vi "Add Channel.vi"(7 "Display State In":T1={"Current Channels Info"=[], "Help Prefix"="", "Max Display Size"=8, "Max Size"=0, "Show Buttons"=TRUE, "Data Valid"=refnum, "Show Range"=FALSE, "Range Items"=[], "Range Index"=[]}, 11 "Channels In":T4) -> (3 "Channels Out":T4, 5 "Display State Out":T1={"Current Channels Info"=[], "Help Prefix"="", "Max Display Size"=8, "Max Size"=0, "Show Buttons"=TRUE, "Data Valid"=refnum, "Show Range"=FALSE, "Range Items"=[], "Range Index"=[]})   [LabVIEW 2021, in "myRIO Channel List.xctl"]
uses:
  <vilib>/myRIO/Common/Express VI Framework/xctls/myRIO Channel List/myRIO Channel List.xctl
  <vilib>/myRIO/Common/Express VI Framework/xctls/myRIO Channel List/Data.ctl
  <vilib>/myRIO/Common/Express VI Framework/xctls/myRIO Channel List/typedefs/Channel Data.ctl
  <vilib>/myRIO/Common/Express VI Framework/xctls/myRIO Channel List/typedefs/Remove Channel.ctl
  <vilib>/myRIO/Common/Express VI Framework/xctls/myRIO Channel List/State.ctl
  <vilib>/myRIO/Common/Profile Manager Framework/typedefs/Channel Info.ctl
  <vilib>/myRIO/Common/Express VI Framework/typedefs/Data Validate Ref.ctl
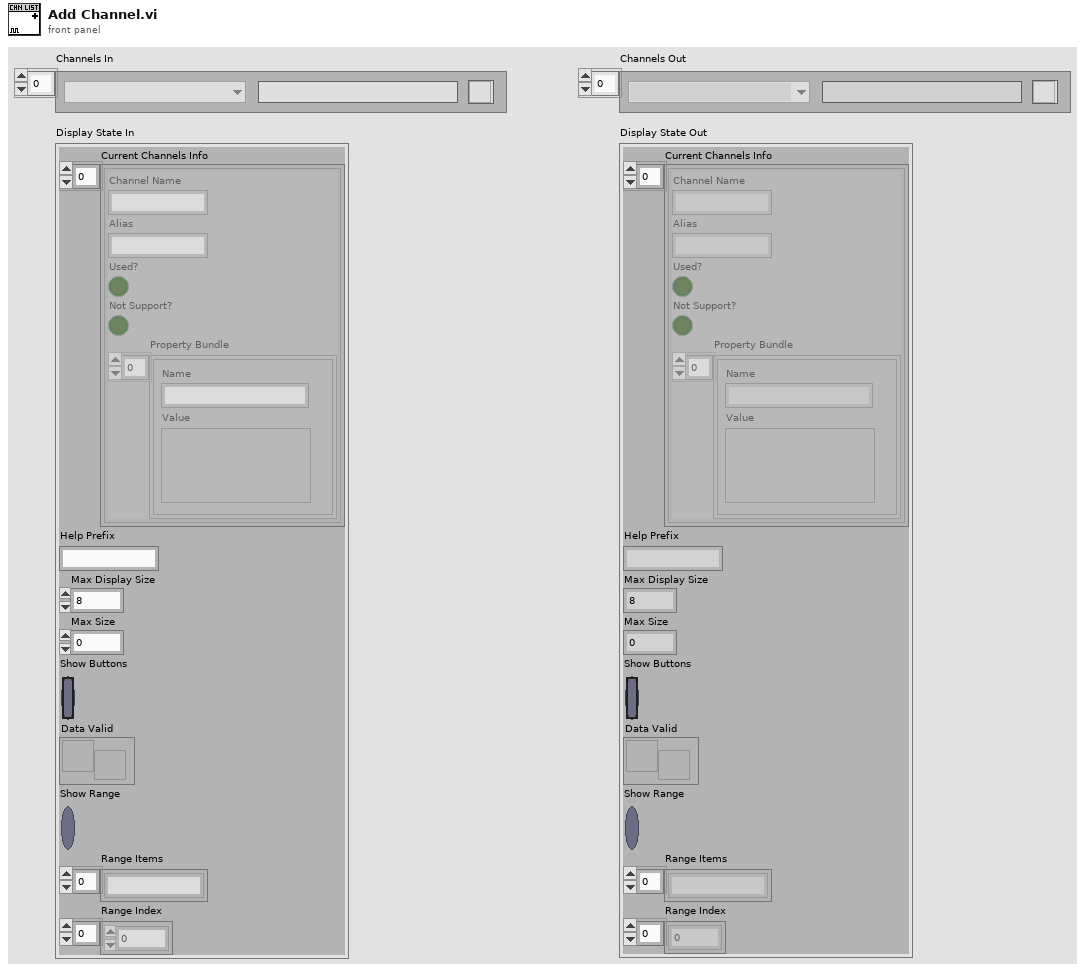
[diagram p1: front panel]
types:
  T1 = typedef "myRIO Channel List.xctl/State.ctl" = cluster{"Current Channels Info":T2[], "Help Prefix":string, "Max Display Size":i32, "Max Size":i32, "Show Buttons":bool, "Data Valid":T3, "Show Range":bool, "Range Items":string[], "Range Index":i32[]}
  T2 = typedef "Channel Info.ctl" = cluster{"Channel Name":string, "Alias":string, "Used?":bool, "Not Support?":bool, "Property Bundle":cluster{"Name":string, "Value":variant}[]}
  T3 = typedef "Data Validate Ref.ctl" = refnum<user-event>
  T4 = typedef "myRIO Channel List.xctl/Data.ctl" = T5[]
  T5 = typedef "myRIO Channel List.xctl/Channel Data.ctl" = cluster{"Channel Name":u16, "Channel Alias":string, "Remove Channel":T6, "Index":i32}
  T6 = typedef "myRIO Channel List.xctl/Remove Channel.ctl" = bool
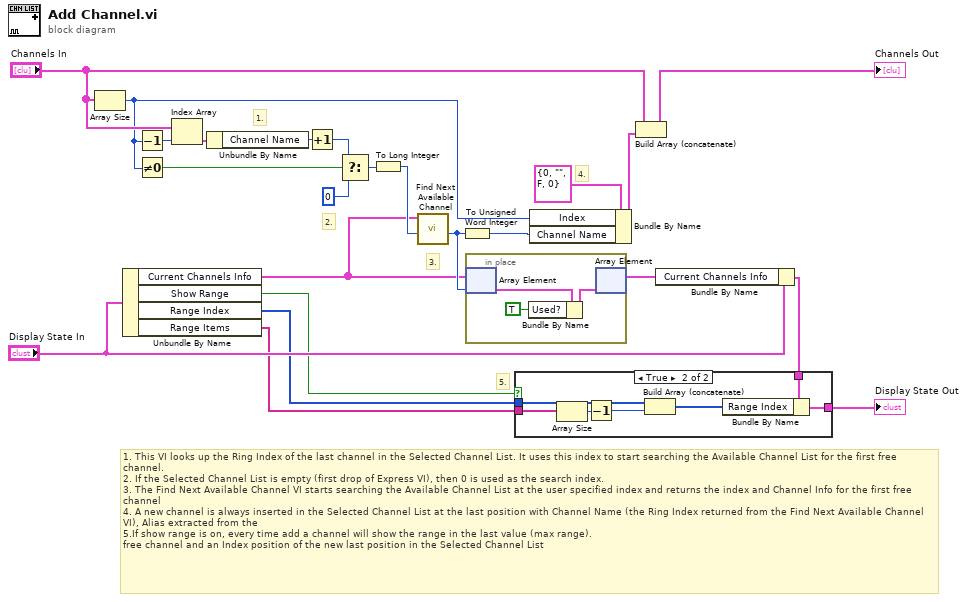
[diagram p0: block diagram]
diagram:
  # "5."
  # "4."
  # "3."
  # "2."
  # "1."
  # "1. This VI looks up the Ring Index of the last channel in the Selected Channel List. It uses this index to start searching the Available Channel List for the first free channel.\n2. If the Selected Channel List is empty (first drop of Express VI), then 0 is used as the search index. \n3. The Find Next Available Channel VI starts searching the Available Channel List at the user specified index and returns the index and Channel Info for the first free channel\n4. A new channel is always inserted in the Selected Channel List at the last position with Channel Name (the Ring Index returned from the Find Next Available Channel VI), Alias extracted from the\n5.If show range is on, every time add a channel will show the range in the last value (max range). \nfree channel and an Index position of the new last position in the Selected Channel List"
  n1 = Array Size(array="Channels In") -> (size(s)=w11:i32)
  n2 = Unbundle By Name("Display State In") -> ("Current Channels Info"=w9:T2[], "Show Range"=w6:bool, "Range Index"=w5:i32[], "Range Items"=w1:string[])
  n3 = Decrement(x=w11) -> (x-1=w14:i32)
  n4 = Not Equal To 0?(x=w11) -> (x != 0?=w2:bool)
  n5 = Index Array(array="Channels In", index=w14) -> (element=w22:T5)
  n6 = Unbundle By Name(w22) -> ("Channel Name"=w21:u16)
  n7 = Increment(x=w21) -> (x+1=w20:u16)
  n8 = Select(t=w20, s=w2, f=u16 0) -> (s? t:f=w18:u16)
  n9 = To Long Integer(number=w18) -> (32bit integer=w17:i32)
  n10 = call <vilib>:"Find Next Available Channel.vi"("Starting Index (0)"=w17, "Channels Info"=w9) -> ("Available Channel Index"=w15:i32)  [unwired: 8 in, 1 out]
  n11 = To Unsigned Word Integer(number=w15) -> (unsigned 16bit integer=w13:u16)
  n12 = in-place {
    n13 = in-place-array #1(w9, w15) -> (w26:T2)
    n14 = Bundle By Name(cluster=w26, "Used?"=TRUE) -> (w25:T2)
    n15 = in-place-array #1(w25) -> (w7:T2[])  [unwired: 1 out]
  }
  n16 = Bundle By Name(cluster=T5 {"Channel Name"=0, "Channel Alias"="", "Remove Channel"=FALSE, "Index"=0} ("Channel"), "Index"=w11, "Channel Name"=w13) -> (w10:T5)
  n17 = Build Array (concatenate)("Channels In", w10) -> (→"Channels Out":T4)
  n18 = Bundle By Name(cluster="Display State In", "Current Channels Info"=w7) -> (w4:T1)
  n19 = case shown="True" w6 {
    tunnel: w1 -> [_ w33]
    tunnel: w5 -> [_ w30]
    tunnel: w4 -> [w27 w32]
    tunnel: [w27 w31] -> w3
    frame False {
    }
    frame True {
      n20 = Array Size(array=w33) -> (size(s)=w34:i32)
      n21 = Decrement(x=w34) -> (x-1=w29:i32)
      n22 = Build Array (concatenate)(w30, w29) -> (w28:i32[])
      n23 = Bundle By Name(cluster=w32, "Range Index"=w28) -> (w31:T1)
    }
  }
  "Display State Out" <- w3
